vi "Actor Core.vi"(8 "error in":errorcluster, 11 "Beta View In":refnum<class "Beta View.lvclass">) -> (0 "error out":errorcluster, 3 "Actor out":refnum<class "Actor.lvclass">)   [LabVIEW 2017, in "Beta View.lvclass"]
doc: "(<B>Filename</B>: Actor Framework.lvlib:Actor.lvclass:Actor Core.vi)\n\nReceives messages to the actor, reacts to them, and initiates any error handling that may shut the actor down.\n\nDescendant classes may override this VI to append parallel tasks for the actor to complete while it handles messages. Overrides use the Call Parent Method node.\n\n<License>\nCopyright © 2017 Composed Systems, LLC | All rights reserved\nwww.composed.io\n\nAuthor: Ethan Stern <ethan.stern@composed.io>\n\nThis software is provided \"AS IS\" WITHOUT WARRANTIES, either express or implied, AND IS FOR EDUCATIONAL PURPOSES ONLY.\n</License>"
uses:
  <vilib>/gpm_packages/@cs/popup-viewmanager/Example/Beta View/Beta View.lvclass
  C:/Program Files/National Instruments/LabVIEW 2017/vi.lib/gpm_packages/@cs/mva-viewable/Source/IViewable/IViewable/IViewable.lvclass
  <vilib>/ActorFramework/Actor/Actor.lvclass
  <vilib>/gpm_packages/@cs/popup-viewmanager/Example/Beta View/Beta View.lvclass/Beta View.ctl
  <vilib>/gpm_packages/@cs/mva-viewable/Source/IViewable/IViewable/IViewable.lvclass
panel:
  out "Ready":string
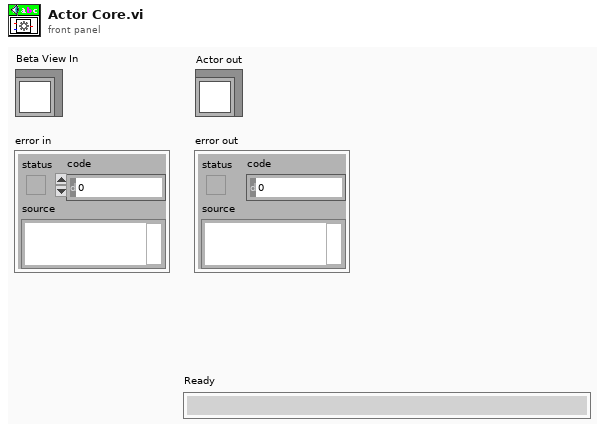
[diagram p1: front panel]
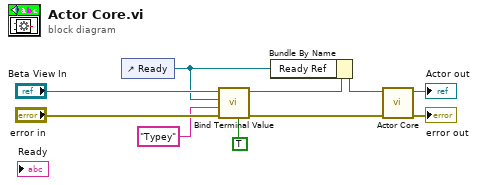
[diagram p0: block diagram]
diagram:
  n1 = control-ref of="Ready"() -> (w2:refnum<vi>)
  n2 = call <vilib>:"Bind Terminal Value.vi"("Ignore Past Updates? (F)"=TRUE, "error in (no error)"="error in", "Datum Name (\"\"=Use Control Label)"="Typey" ("Datum Name (\"\"=Use Control Label)"), "Ctl Refnum"=w2, "IViewable in"="Beta View In") -> ("error out"=w6:errorcluster, "IViewable out"=w4:refnum<class "Beta View.lvclass">)  [unwired: 5 in]
  n3 = Bundle By Name(cluster=w4, "Ready Ref"=w2) -> (w3:refnum<class "Beta View.lvclass">)
  n4 = call-parent "Actor Core.vi"("error in"=w6, "IViewable In"=w3) -> ("error out"=→"error out":errorcluster, "Actor out"=→"Actor out":refnum<class "Actor.lvclass">)  [unwired: 8 in]
